vi "PaternSolve2.vi"(4 "orange":string[](array[string]), 6 "jaune":string[](array[string]), 8 "Vert":string[](array[string]), 9 "white":string[](array[string]), 10 "rouge":string[](array[string]), 11 "bleu":string[](array[string])) -> (3 "RubixTab solver":string[][](array[string]))   [LabVIEW 2019]
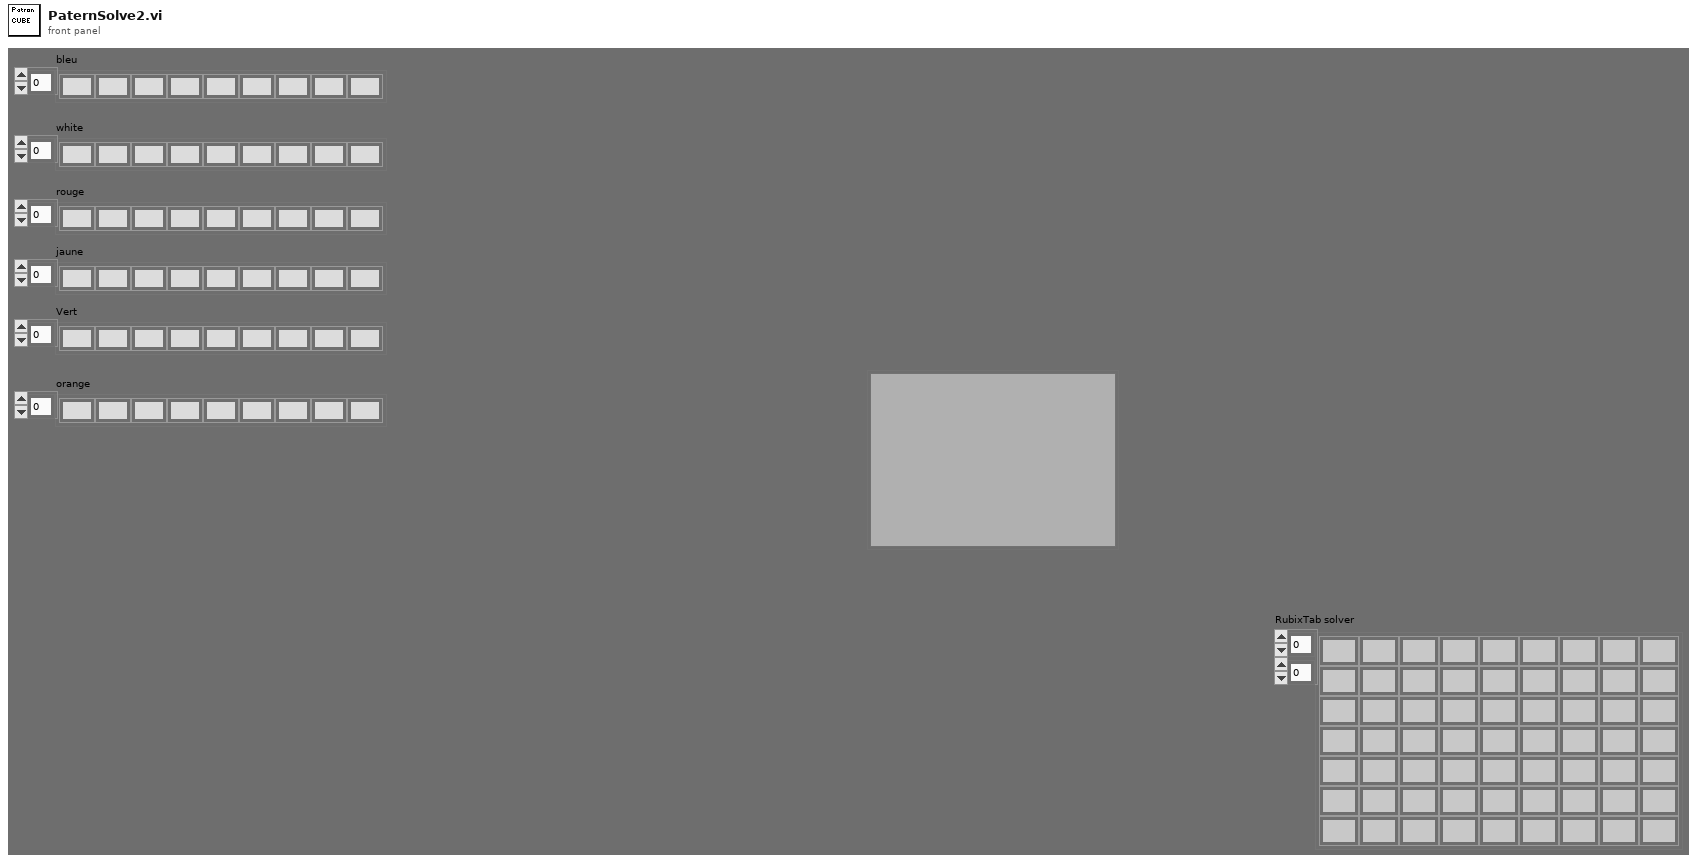
[diagram p1: front panel]
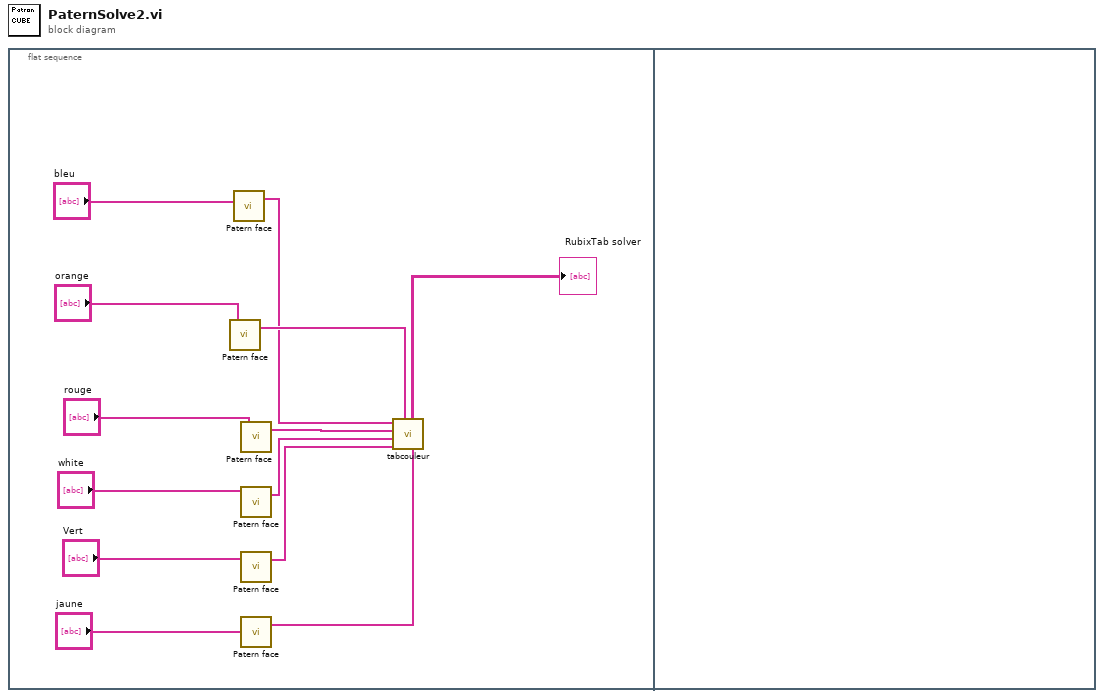
[diagram p0: block diagram]
diagram:
  n1 = flat-sequence {
    frame #0 {
      n2 = call "Patern face.vi"("Array"="orange") -> ("Final array"=w11:string[])  [unwired: 18 in]
      n3 = call "Patern face.vi"("Array"="bleu") -> ("Final array"=w7:string[])  [unwired: 18 in]
      n4 = call "Patern face.vi"("Array"="rouge") -> ("Final array"=w8:string[])  [unwired: 18 in]
      n5 = call "Patern face.vi"("Array"="white") -> ("Final array"=w9:string[])  [unwired: 18 in]
      n6 = call "Patern face.vi"("Array"="Vert") -> ("Final array"=w10:string[])  [unwired: 18 in]
      n7 = call "Patern face.vi"("Array"="jaune") -> ("Final array"=w12:string[])  [unwired: 18 in]
      n8 = call "tabcouleur.vi"("Blue"=w7, "Red"=w8, "White"=w9, "Green"=w10, "Orange"=w11, "Yellow"=w12) -> ("RubixTab solver"=→"RubixTab solver":string[][])  [unwired: 4 in]
    }
    frame #1 {
    }
  }
